vi "Read FunctionCreateFileHandler.vi"(8 "error in (no error)":errorcluster, 11 "LoggingWrapper in":refnum<class "LoggingWrapper.lvclass">) -> (0 "error out":errorcluster, 2 "FunctionCreateFileHandler":string, 3 "LoggingWrapper out":refnum<class "LoggingWrapper.lvclass">)   [LabVIEW 2022 SP3, in "Logger.lvlib" / "LoggingWrapper.lvclass"]
uses:
  LoggingWrapper.lvclass
  LoggingWrapper.lvclass/LoggingWrapper.ctl
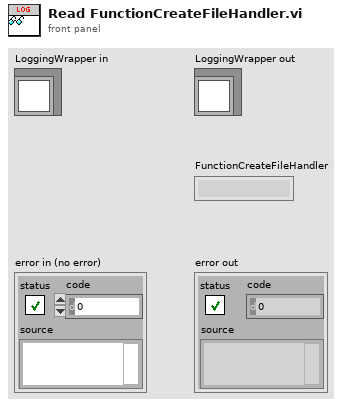
[diagram p1: front panel]
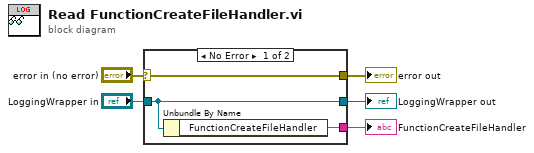
[diagram p0: block diagram]
diagram:
  n1 = case shown="No Error" "error in (no error)" {
    selector: "error in (no error)" -> [w8 w9]
    tunnel: [w8 w9] -> w4
    tunnel: [w7 w10] -> w2
    tunnel: "LoggingWrapper in" -> [w7 w10]
    tunnel: [w6 _] -> w1
    frame No Error {
      n2 = Unbundle By Name(w7) -> ("FunctionCreateFileHandler"=w6:string)
    }
    frame Error {
    }
  }
  "error out" <- w4
  "LoggingWrapper out" <- w2
  "FunctionCreateFileHandler" <- w1
